vi "getAllUnrestrictedChannels.vi"(8 "error in (no error)":errorcluster, 11 "DeviceArray in":refnum<class "DeviceArray.lvclass">) -> (0 "error out":errorcluster, 2 "ChannelArray.lvclass":refnum<class "ChannelArray.lvclass">, 3 "DeviceArray out":refnum<class "DeviceArray.lvclass">)   [LabVIEW 2009, in "Tools.lvlib" / "DatabaseHelpers.lvlib" / "DeviceArray.lvclass"]
uses:
  DeviceArray.lvclass
  ChannelArray/ChannelArray.lvclass
  DeviceArray.lvclass/DeviceArray.ctl
  device/device.lvclass
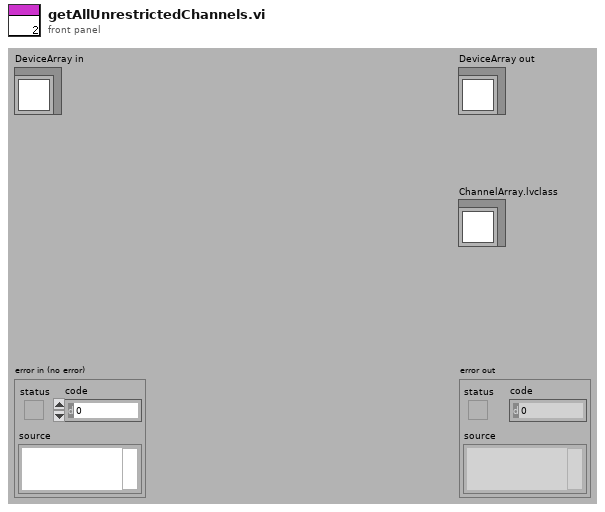
[diagram p1: front panel]
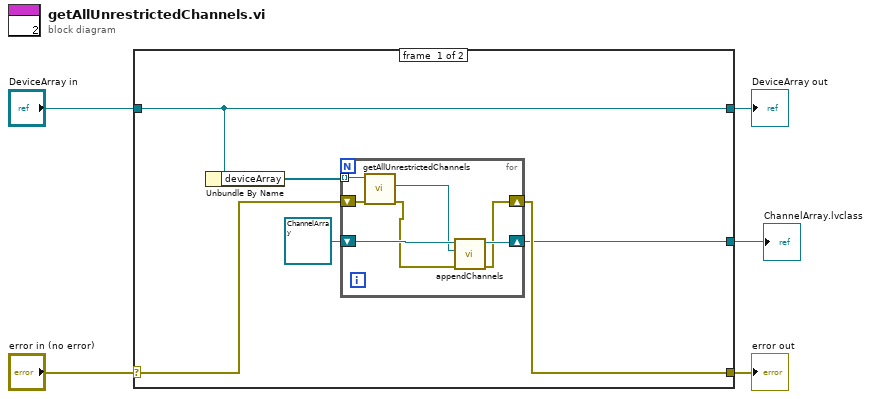
[diagram p0: block diagram]
diagram:
  n1 = case shown="No Error" "error in (no error)" {
    selector: "error in (no error)" -> [w8 w20]
    tunnel: [w7 w20] -> w4
    tunnel: [w11 w19] -> w2
    tunnel: "DeviceArray in" -> [w11 w19]
    tunnel: [w6 _] -> w1
    frame #0 {
      n2 = Unbundle By Name(w11) -> ("deviceArray"=w10:refnum<class "device.lvclass">[])
      n3 = for {
        tunnel: w10 -> [w15] mode=indexing
        shift-right: [w17] -> w6
        shift-left: refnum<class "ChannelArray.lvclass"> refnum ("ChannelArray out") -> [w18]
        shift-right: [w16] -> w7
        shift-left: w8 -> [w12]
        n4 = call "getAllUnrestrictedChannels.vi"("error in (no error)"=w12, "device in"=w15) -> ("error out"=w13:errorcluster, "ChannelArray.lvclass"=w14:refnum<class "ChannelArray.lvclass">)  [unwired: 7 in, 1 out]
        n5 = call "appendChannels.vi"("error in (no error)"=w13, "ChannelArrayToAppend"=w14, "ChannelArray in"=w18) -> ("error out"=w16:errorcluster, "ChannelArray out"=w17:refnum<class "ChannelArray.lvclass">)  [unwired: 7 in]
      }
    }
    frame #1 {
    }
  }
  "error out" <- w4
  "DeviceArray out" <- w2
  "ChannelArray.lvclass" <- w1
